vi "Update ring names.vi"(8 "error in (no error)":errorcluster, 9 "Update from File-group-channel":bool, 10 "Names Array":string[](array[string]), 11 "MagLabGraph in":refnum<class "XY Plot.lvclass">) -> (0 "error out":errorcluster, 3 "MagLabGraph out":refnum<class "XY Plot.lvclass">)   [LabVIEW 2015, in "XY Plot.lvclass"]
uses:
  XY Plot.lvclass
  XY Plot.lvclass/XY Plot.ctl
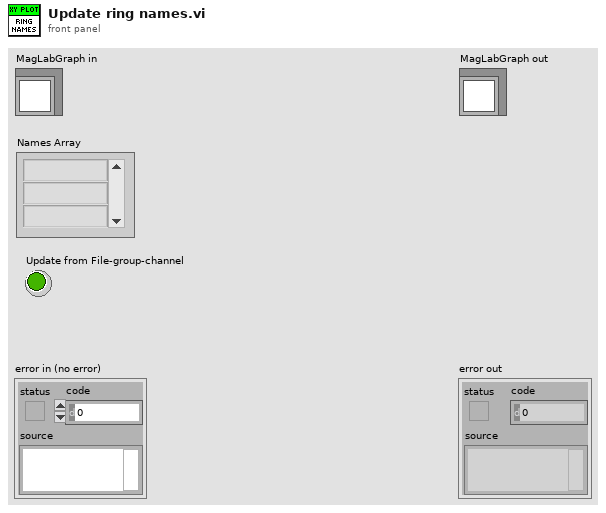
[diagram p1: front panel]
types:
  T1 = cluster{"File Path Control":path, "Group":string, "Channel":string, "Abbreviated":string}[]
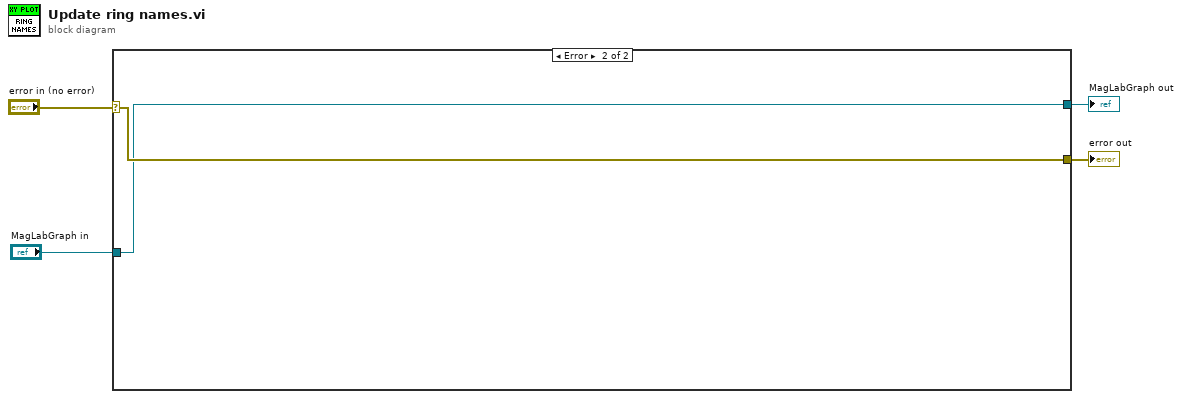
[diagram p0: block diagram]
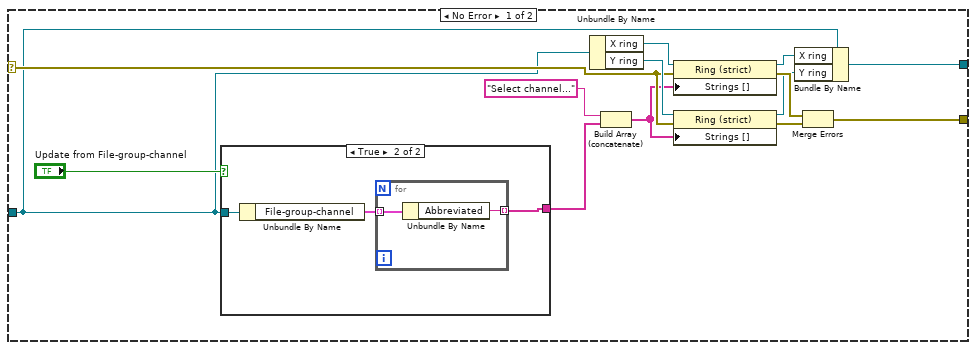
[diagram p2: hidden frame]
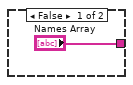
[diagram p3: hidden frame]
diagram:
  n1 = case shown="Error" "error in (no error)" {
    selector: "error in (no error)" -> [w16 w26]
    tunnel: [w10 w26] -> w3
    tunnel: [w9 w25] -> w1
    tunnel: "MagLabGraph in" -> [w5 w25]
    frame No Error {
      n2 = case shown="True" "Update from File-group-channel" {
        tunnel: ["Names Array" w20] -> w15
        tunnel: w5 -> [_ w22]
        frame False {
        }
        frame True {
          n3 = Unbundle By Name(w22) -> ("File-group-channel"=w21:T1)
          n4 = for {
            tunnel: w21 -> [w24] mode=indexing
            tunnel: [w23] -> w20 mode=indexing
            n5 = Unbundle By Name(w24) -> ("Abbreviated"=w23:string)
          }
        }
      }
      n6 = Unbundle By Name(w5) -> ("X ring"=w18:refnum<vi>, "Y ring"=w17:refnum<vi>)
      n7 = Build Array (concatenate)("Select channel...", w15) -> (w13:string[])
      n8 = property class="Ring (strict)"(reference=w18, error in=w16, "Strings []"=w13) -> (reference out=w8:refnum<vi>, error out=w12:errorcluster)
      n9 = property class="Ring (strict)"(reference=w17, error in=w16, "Strings []"=w13) -> (reference out=w7:refnum<vi>, error out=w11:errorcluster)
      n10 = Bundle By Name(cluster=w5, "X ring"=w8, "Y ring"=w7) -> (w9:refnum<class "XY Plot.lvclass">)
      n11 = Merge Errors(w12, w11) -> (w10:errorcluster)
    }
    frame Error {
    }
  }
  "error out" <- w3
  "MagLabGraph out" <- w1
